vi "动力环境监测系统.vi"() -> ()   [LabVIEW 2016, in "环境动力监测库.lvlib"]
panel:
  in  "单选按钮":enum32{"自动重合闸", "电源管理", "仪器电源管理"}(radio)
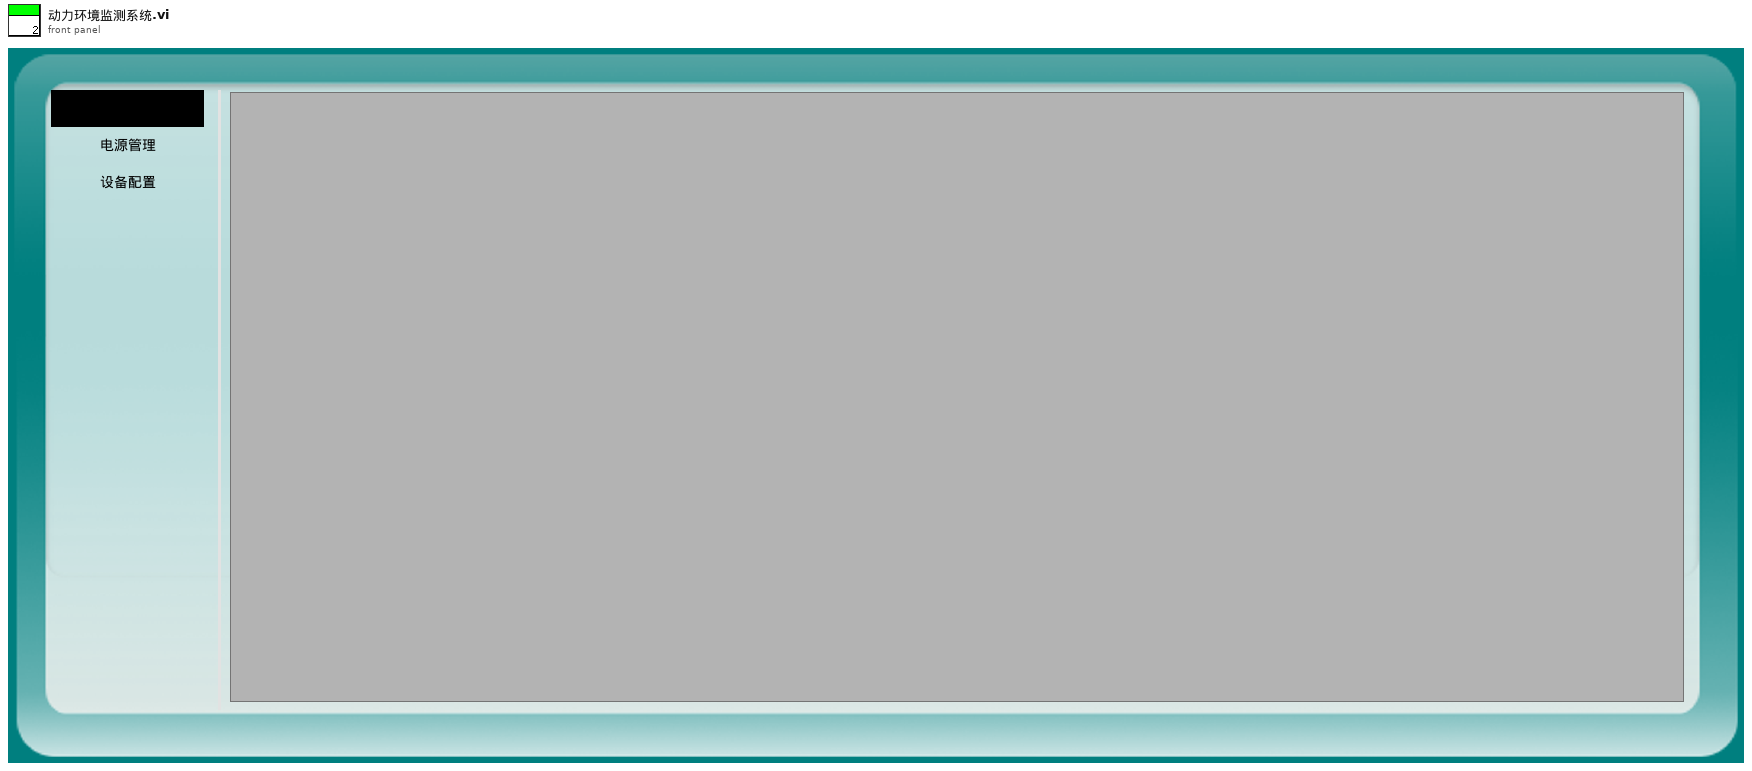
[diagram p1: front panel]
types:
  T1 = enum32{"Bad", "Idle", "Run top level", "Running"}
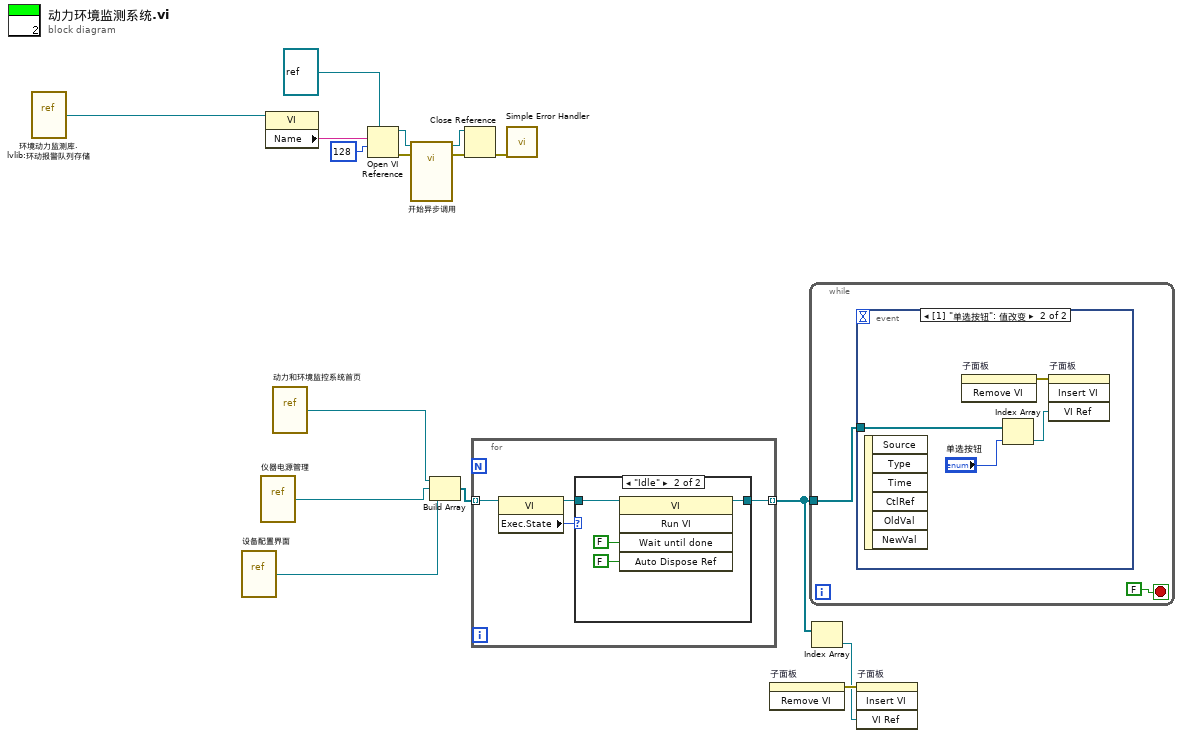
[diagram p0: block diagram]
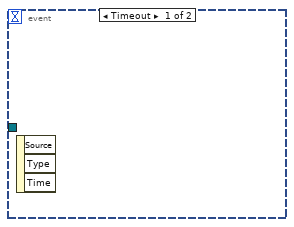
[diagram p2: hidden frame]
diagram:
  n1 = vi-ref "环境动力监测库.lvlib:环动报警队列存储.vi"() -> (w7:refnum<vi>)
  n2 = vi-ref "设备配置界面.vi"() -> (w10:refnum<vi>)
  n3 = vi-ref "仪器电源管理.vi"() -> (w11:refnum<vi>)
  n4 = property class="VI"(reference=w7) -> ("Name"=w6:string)  [unwired: 1 in, 2 out]
  n5 = vi-ref "动力和环境监控系统首页.vi"() -> (w12:refnum<vi>)
  n6 = Open VI Reference(type specifier VI Refnum (for type only)=refnum<vi> refnum ("类型说明符VI引用句柄（仅用于类型）"), vi path=w6, options=128 ("选项")) -> (vi reference=w4:refnum<vi>, error out=w8:errorcluster)  [unwired: 3 in]
  n7 = call-by-ref "开始异步调用"(reference=w4, error in=w8) -> (reference out=w3:refnum<vi>, error out=w2:errorcluster)  [unwired: 12 in]
  n8 = Build Array(w12, w11, w10) -> (w16:refnum<vi>[])
  n9 = Close Reference(reference=w3, error in (no error)=w2) -> (error out=w1:errorcluster)
  n10 = for {
    tunnel: w16 -> [w20] mode=indexing
    tunnel: [w17] -> w13 mode=indexing
    n11 = property class="VI"(reference=w20) -> (reference out=w18:refnum<vi>, "Exec.State"=w19:T1)  [unwired: 1 in, 1 out]
    n12 = case shown="\"Idle\"" w19 {
      tunnel: w18 -> [w21 w23]
      tunnel: [w21 w22] -> w17
      frame "Bad", Default {
      }
      frame "Idle" {
        n13 = invoke class="VI" method="Run VI"(reference=w23, "Wait until done"=FALSE ("结束前等待"), "Auto Dispose Ref"=FALSE ("自动销毁引用")) -> (reference out=w22:refnum<vi>)  [unwired: 2 in, 4 out]
      }
    }
  }
  n14 = call <vilib>:"Simple Error Handler.vi"("error in (no error)"=w1) -> ()  [unwired: 4 in, 5 out]
  n15 = invoke on="子面板" class="SubPnl" method="Remove VI"() -> (error out=w15:errorcluster)  [unwired: 3 in, 2 out]
  n16 = while {
    tunnel: w13 -> [w26]
    stop <- FALSE stop-if-true
    n17 = event shown="[1] \"单选按钮\": 值改变" {
      selector: _ -> [_ _]
      dyn-events: _ -> [_ _]
      timeout: _ -> [_ _]
      tunnel: w26 -> [_ w29]
      event Timeout {
        n18 = event-data() -> ()  [unwired: 1 in, 3 out]
      }
      event "单选按钮": Value Change {
        n19 = event-data() -> ()  [unwired: 1 in, 6 out]
        n20 = invoke on="子面板" class="SubPnl" method="Remove VI"() -> (error out=w31:errorcluster)  [unwired: 3 in, 2 out]
        n21 = Index Array(array=w29, index="单选按钮") -> (element=w30:refnum<vi>)
        n22 = invoke on="子面板" class="SubPnl" method="Insert VI"(error in=w31, "VI Ref"=w30) -> ()  [unwired: 2 in, 4 out]
      }
    }
  }
  n23 = Index Array(array=w13) -> (element=w14:refnum<vi>)  [unwired: 1 in]
  n24 = invoke on="子面板" class="SubPnl" method="Insert VI"(error in=w15, "VI Ref"=w14) -> ()  [unwired: 2 in, 4 out]
